vi "VoltDecode-AdvMultiRec.vi"(4 "Adj.SegmentSize":dbl=4.0, 5 "Offset":sgl, 6 "Adj.Depth":dbl=4.0, 7 "Slope":sgl=1.0, 8 "Depth":dbl=4.0, 9 "Channels":i32=1, 10 "cSegment":i32, 11 "Buffer In":u8[](array[numeric])) -> (2 "Data (V)":sgl[](array[numeric]) format="%.2f", 3 "Buffer Out":u8[](array[numeric]))   [LabVIEW 2014]
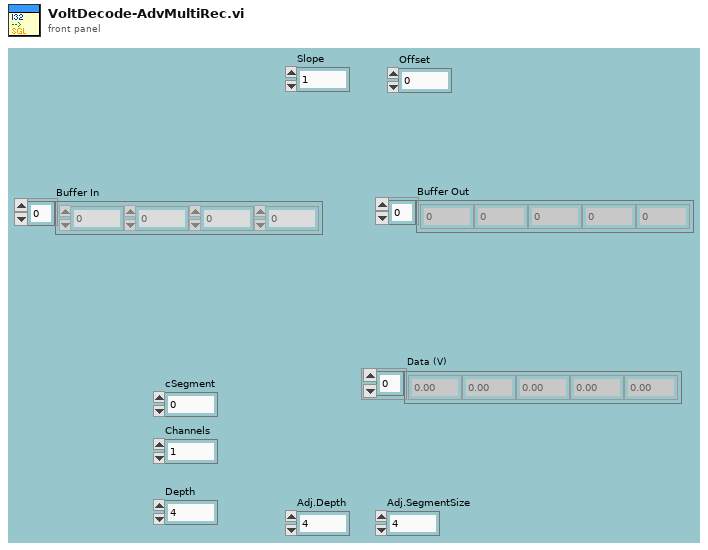
[diagram p1: front panel]
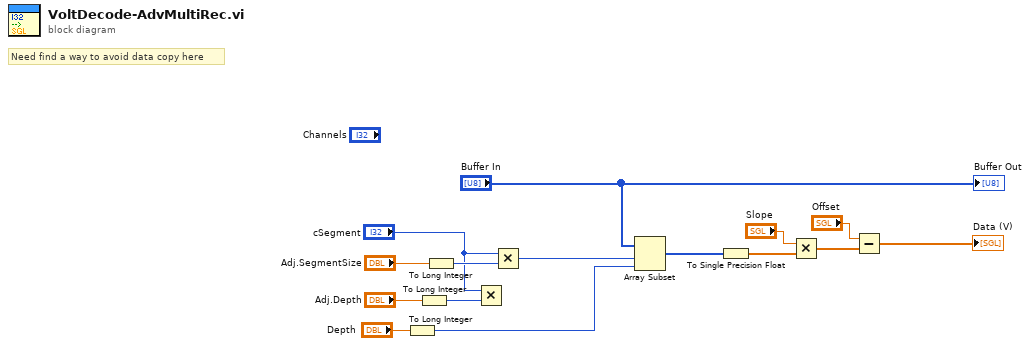
[diagram p0: block diagram]
diagram:
  # "Need find a way to avoid data copy here"
  n1 = To Long Integer(number="Depth") -> (32bit integer=w6:i32)
  n2 = To Long Integer(number="Adj.Depth") -> (32bit integer=w11:i32)
  n3 = To Long Integer(number="Adj.SegmentSize") -> (32bit integer=w12:i32)
  n4 = Multiply(x="cSegment", y=w11) -> ()  [unwired: 1 out]
  n5 = Multiply(x="cSegment", y=w12) -> (x*y=w10:i32)
  n6 = Array Subset(array="Buffer In", index=w10, length=w6) -> (w1:u8[])
  n7 = To Single Precision Float(number=w1) -> (single precision float=w4:sgl[])
  n8 = Multiply(x="Slope", y=w4) -> (x*y=w5:sgl[])
  n9 = Subtract(x="Offset", y=w5) -> (x-y=→"Data (V)":sgl[])
  "Buffer Out" <- "Buffer In"
